vi "FindDAQDevice.vi"(0 "Model In":string="USB-TC01", 11 "error in (no error)":errorcluster) -> (4 "DAQmx Device Name":tag, 6 "Model":string, 8 "x = y?":bool, 15 "error out":errorcluster)   [LabVIEW 2018]
uses:
  <resource>/objmgr/daqmx.rc
panel:
  out "Array":string[](array[string])
  out "concatenated string":string
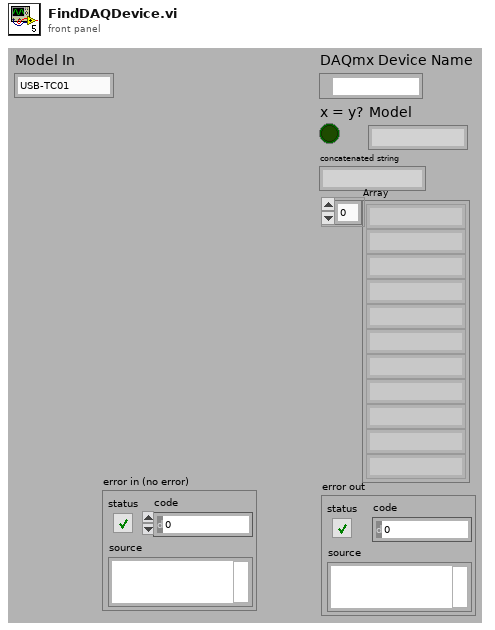
[diagram p1: front panel]
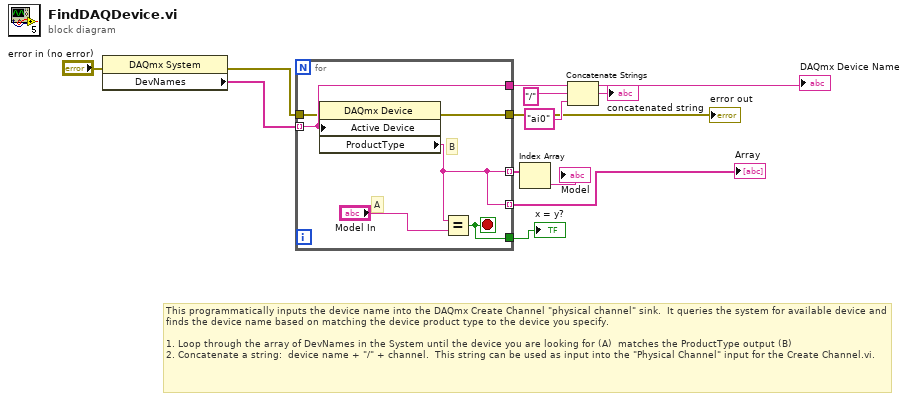
[diagram p0: block diagram]
diagram:
  # "This programmatically inputs the device name into the DAQmx Create Channel \"physical channel\" sink.  It queries the system for available device and finds the device name based on matching the device product type to the device you specify.\n\n1. Loop through the array of DevNames in the System until the device you are looking for (A)  matches the ProductType output (B)\n2. Concatenate a string:  device name + \"/\" + channel.  This string can be used as input into the \"Physical Channel\" input for the Create Channel.vi."
  n1 = property class="DAQmx System"(error in="error in (no error)") -> (error out=w4:errorcluster, "DevNames"=w12:tag[])  [unwired: 1 in, 1 out]
  n2 = for {
    tunnel: w12 -> [w18] mode=indexing
    tunnel: [w13] -> w7 mode=indexing
    tunnel: [w18] -> w11
    tunnel: [w16] -> w6
    tunnel: w4 -> [w15]
    tunnel: [w14] -> w3
    tunnel: [w13] -> w1 mode=indexing
    stop <- w16 stop-if-true
    # "B"
    # "A"
    n3 = property class="DAQmx Device"(error in=w15, "Active Device"=w18) -> (error out=w14:errorcluster, "ProductType"=w13:string)  [unwired: 1 in, 1 out]
    n4 = Equal?(x=w13, y="Model In") -> (x = y?=w16:bool)
  }
  "Array" <- w1
  "DAQmx Device Name" <- w11
  "x = y?" <- w6
  "error out" <- w3
  n5 = Index Array(array=w7) -> (element=→"Model":string)  [unwired: 1 in]
  n6 = Concatenate Strings(w11, "/" ("string"), "ai0" ("string")) -> (→"concatenated string":string)
